vi "globalTearDown.vi"(8 "error in (no error)":errorcluster, 11 "testcase-CSMSubModule in":refnum<class "testcase-CSMSubModule.lvclass">) -> (0 "error out":errorcluster, 3 "testcase-CSMSubModule out":refnum<class "testcase-CSMSubModule.lvclass">)   [LabVIEW 2017, in "testcase-CSMSubModule.lvclass"]
uses:
  testcase-CSMSubModule.lvclass
  testcase-CSMSubModule.lvclass/testcase-CSMSubModule.ctl
  <vilib>/addons/_JKI Toolkits/VI Tester/TestCase.llb/TestCase.lvclass
  src/user.lib/_NEVSTOP/Communicable State Machine(CSM)/_Support/Typedef/_CSM_List Module Scope.ctl
  src/user.lib/_NEVSTOP/Communicable State Machine(CSM)/Communicable State Machine.lvlib
panel:
  out "CSMs":string[](array[string])
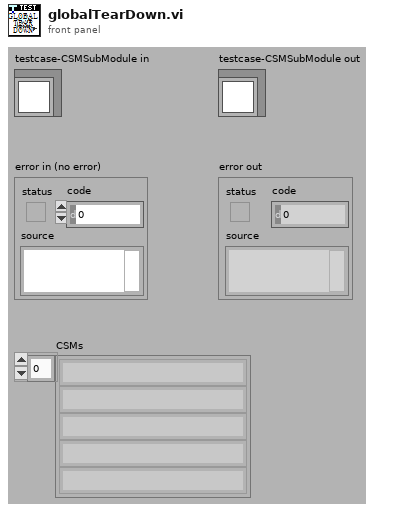
[diagram p1: front panel]
types:
  T1 = typedef "Communicable State Machine.lvlib/_CSM_List Module Scope.ctl" = enum16{"Normal", "System Only", "All"}
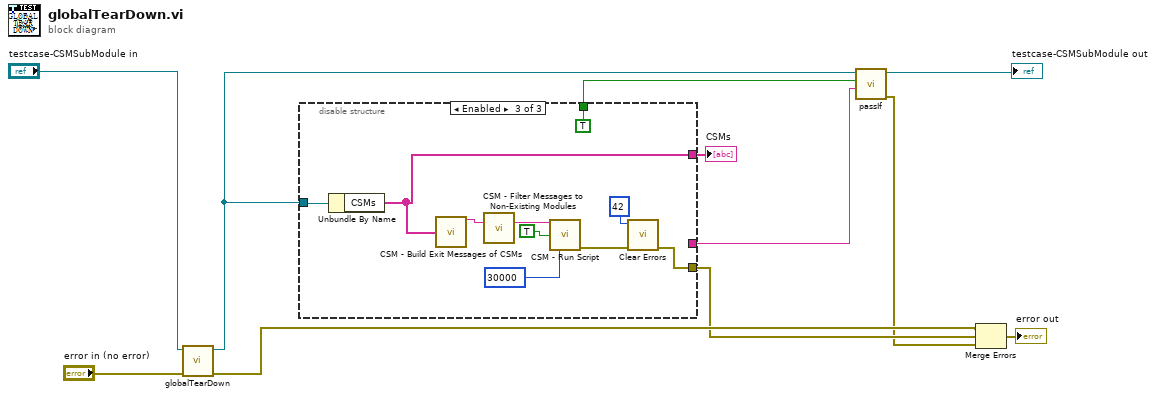
[diagram p0: block diagram]
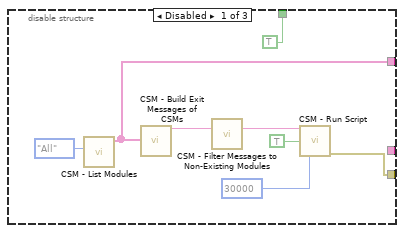
[diagram p2: hidden frame]
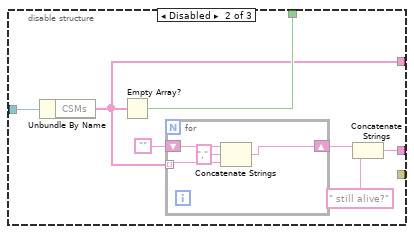
[diagram p3: hidden frame]
diagram:
  n1 = call-parent "globalTearDown.vi"("error in (no error)"="error in (no error)", "TestCase in"="testcase-CSMSubModule in") -> ("error out"=w6:errorcluster, "TestCase out"=w2:refnum<class "testcase-CSMSubModule.lvclass">)  [unwired: 8 in]
  n2 = disable-structure shown="Enabled" {
    disable-tunnel: [w15 _ w33] -> w5
    disable-tunnel: w2 -> [_ w26 w40]
    disable-tunnel: [w14 w24 w36] -> w1
    disable-tunnel: [TRUE w25 TRUE ("pass")] -> w8
    disable-tunnel: [_ w20 _] -> w7
    frame Disabled {
      n3 = call "CSM - List Modules.vi"("Scope (Normal)"=_CSM_List_Module_Scope."All") -> ("Module Names"=w14:string[])  [unwired: 9 in, 1 out]
      n4 = call "CSM - Build Exit Messages of CSMs.vi"("CSMs"=w14) -> ("States"=w19:string)  [unwired: 14 in]
      n5 = call "CSM - Filter Messages to Non-Existing Modules.vi"("States In"=w19) -> ("States Out"=w17:string)  [unwired: 14 in]
      n6 = call "CSM - Run Script.vi"("CSM Scripts"=w17, "Continue If Error? (F)"=TRUE, "Response Timeout (-2 Using Global Settings)"=30000) -> ("error out"=w15:errorcluster)  [unwired: 10 in, 2 out]
    }
    frame Disabled {
      n7 = Unbundle By Name(w26) -> ("CSMs"=w24:string[])
      n8 = Empty Array?(array=w24) -> (empty?=w25:bool)
      n9 = for {
        tunnel: w24 -> [w28] mode=indexing
        shift-right: [w29] -> w22
        shift-left: "" -> [w30]
        n10 = Concatenate Strings(w30, "," ("string"), w28) -> (w29:string)
      }
      n11 = Concatenate Strings(w22, " still alive?" ("string")) -> (w20:string)
    }
    frame Enabled {
      n12 = Unbundle By Name(w40) -> ("CSMs"=w36:string[])
      n13 = call "CSM - Build Exit Messages of CSMs.vi"("CSMs"=w36) -> ("States"=w39:string)  [unwired: 14 in]
      n14 = call "CSM - Filter Messages to Non-Existing Modules.vi"("States In"=w39) -> ("States Out"=w37:string)  [unwired: 14 in]
      n15 = call "CSM - Run Script.vi"("CSM Scripts"=w37, "Continue If Error? (F)"=TRUE, "Response Timeout (-2 Using Global Settings)"=30000) -> ("error out"=w35:errorcluster)  [unwired: 10 in, 2 out]
      n16 = call <vilib>:"Clear Errors.vi"("error in (no error)"=w35, "specific error code to clear (0: all)"=42) -> ("error out"=w33:errorcluster)  [unwired: 4 in, 1 out]
    }
  }
  "CSMs" <- w1
  n17 = call-dynamic "passIf.vi"("message (\"\")"=w7, "pass"=w8, "TestCase in"=w2) -> ("error out"=w4:errorcluster, "TestCase out"=→"testcase-CSMSubModule out":refnum<class "testcase-CSMSubModule.lvclass">)  [unwired: 7 in]
  n18 = Merge Errors(w6, w5, w4) -> (→"error out":errorcluster)
